vi "IsEmptyObject.vi"(3 "error in (no error)":errorcluster, 5 "reference in":refnum<class "G#Interface.lvclass">) -> (0 "error out":errorcluster, 1 "is empty?":bool, 2 "reference out":refnum<class "G#Interface.lvclass">)   [LabVIEW 2017, in "G#Interface.lvclass"]
doc: "Checks if the reference is of G#Object type and thereby an empty object."
uses:
  <vilib>/addons/_AddQ/G#Interface/G#Interface.lvclass
  <vilib>/addons/_AddQ/G#Interface/G#Interface.lvclass/G#Interface.ctl
  <vilib>/addons/_AddQ/G#Object/G#Object.lvclass
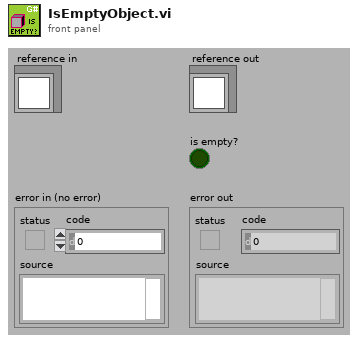
[diagram p1: front panel]
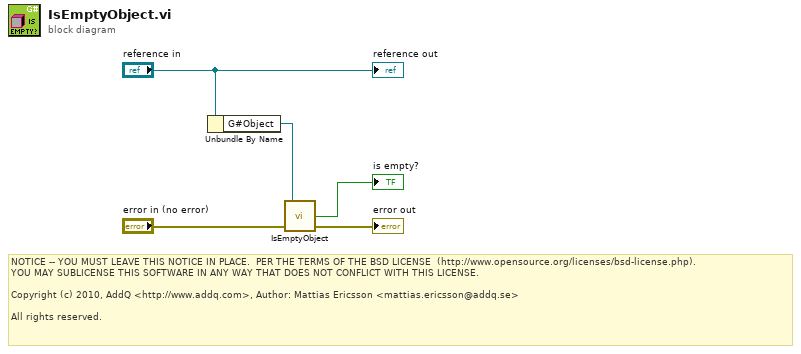
[diagram p0: block diagram]
diagram:
  # "NOTICE -- YOU MUST LEAVE THIS NOTICE IN PLACE.  PER THE TERMS OF THE BSD LICENSE  (http://www.opensource.org/licenses/bsd-license.php).\nYOU MAY SUBLICENSE THIS SOFTWARE IN ANY WAY THAT DOES NOT CONFLICT WITH THIS LICENSE.\n\nCopyright (c) 2010, AddQ <http://www.addq.com>, Author: Mattias Ericsson <mattias.ericsson@addq.se>\n\nAll rights reserved."
  n1 = Unbundle By Name("reference in") -> ("G#Object"=w3:refnum<class "G#Object.lvclass">)
  n2 = call-dynamic "IsEmptyObject.vi"("error in (no error)"="error in (no error)", "reference in"=w3) -> ("error out"=→"error out":errorcluster, "is empty?"=→"is empty?":bool)  [unwired: 1 in, 1 out]
  "reference out" <- "reference in"
